vi "Right Prim.vi"() -> ()   [LabVIEW 2013]
uses:
  Goal.ctl
  <vilib>/Analysis/Matrix/Datatypes/RealMatrix.ctl
  ROS/Code/SubVIs/BaxterSide.ctl
  Baxter Examples/Arm Globals.vi
  <vilib>/Analysis/Matrix/NI_Matrix.lvlib
panel:
  out "Q size 2":i32
  in  "Zero V 2":bool
  in  "L: Home":bool caption="Home"
  in  "L: End":bool caption="Abort"
  in  "L: Pause":bool caption="Pause"
  out "L: Status":string caption="Prim Status"
  out "L: Cmd":cluster{string, "Joints":dbl[]}
  in  "Use Sparse":bool=TRUE
  out "Q size":i32
  in  "Zero V":bool
  in  "R: Home":bool caption="Home"
  in  "R: End":bool caption="Abort"
  in  "R: Pause":bool caption="Pause"
  in  "stop":bool
  out "Status":string caption="Prim Status"
  out "R: Cmd":cluster{string, "Joints":dbl[]}
  # "Right"
  # "Left"
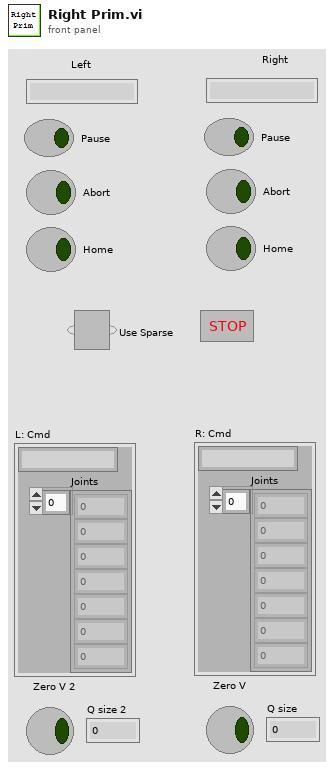
[diagram p1: front panel]
types:
  T1 = typedef "Goal.ctl" = cluster{"Segment":dbl, "T Matrix":T2, "Joints":dbl[], "Label":string, "Joint Motion":bool}
  T2 = typedef "NI_Matrix.lvlib/RealMatrix.ctl" = dbl[][]
  T3 = typedef "BaxterSide.ctl" = enum16{"left", "right"}
  T4 = enum32{"Position", "Velocity", "Effort", "Pause", "Repeat", "End"}
  T5 = typedef "_ROSControl.ctl" = cluster{"topic port":u16, "Node":string, "topic":string, "type":string, "node port":u32, "error ":errorcluster, "Direction":T6, "APIs":string[]}
  T6 = typedef "_ROSDirection.ctl" = enum16{"Node", "Publisher", "Subscriber", "Service Client"}
  T7 = cluster{"Joint Names":string[], "Position":dbl[], "Velocity":dbl[], "Effort":dbl[]}
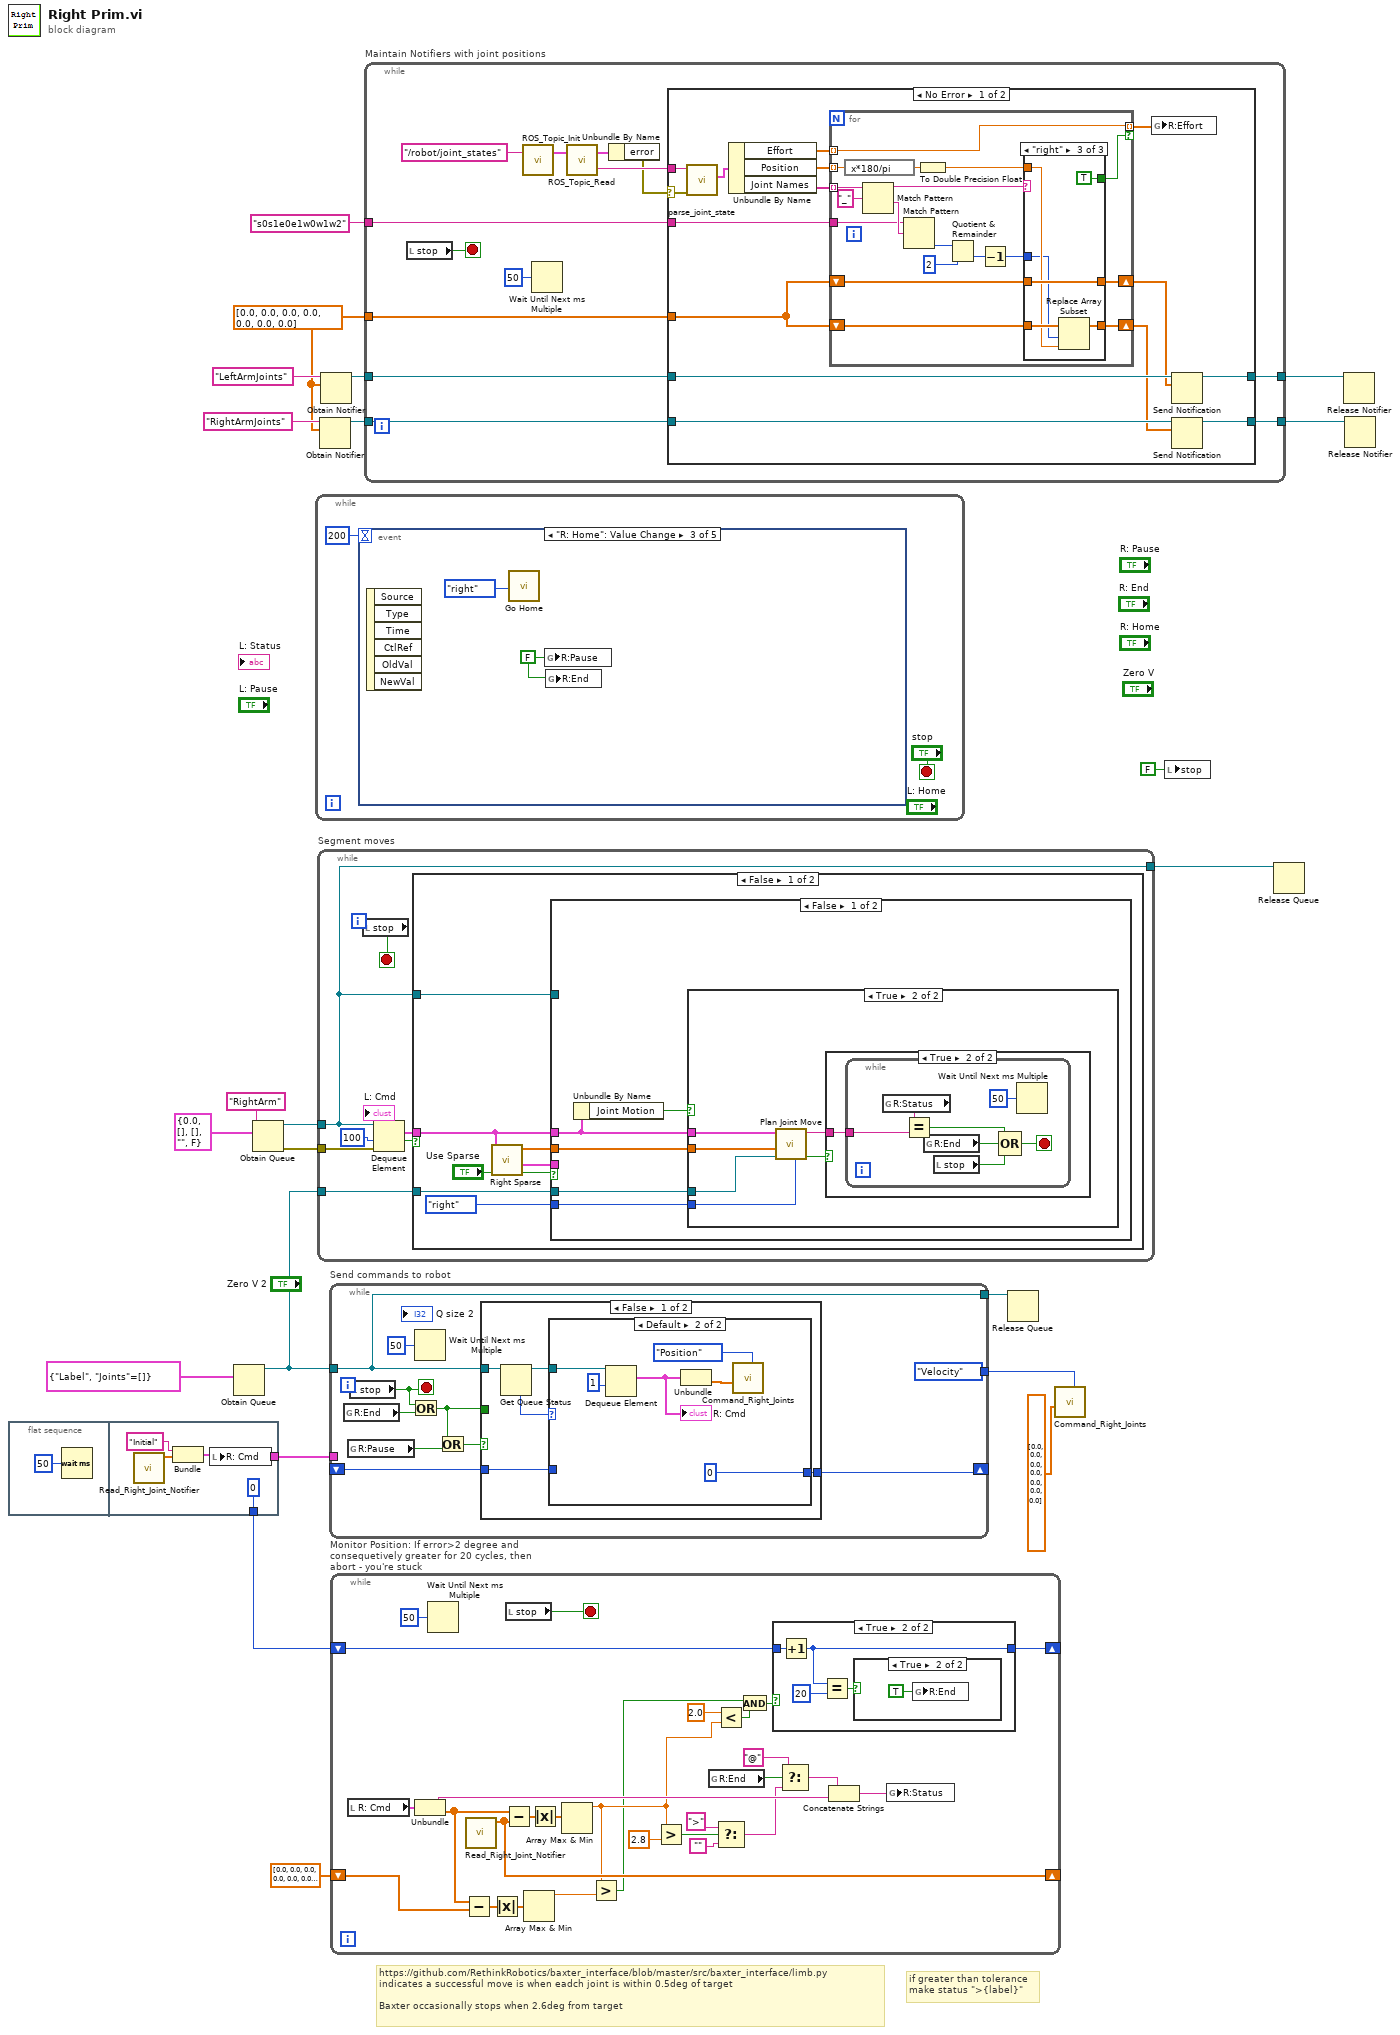
[diagram p0: block diagram]
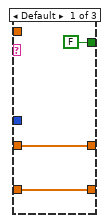
[diagram p2: hidden frame]
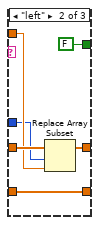
[diagram p3: hidden frame]
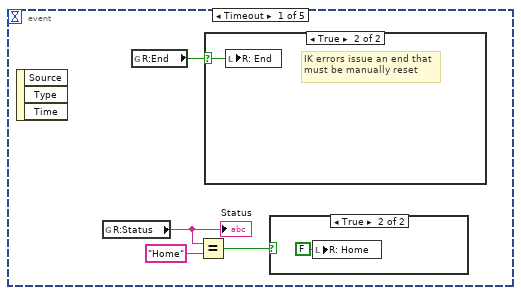
[diagram p5: hidden frame]
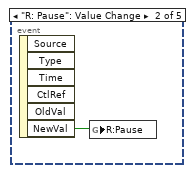
[diagram p8: hidden frame]
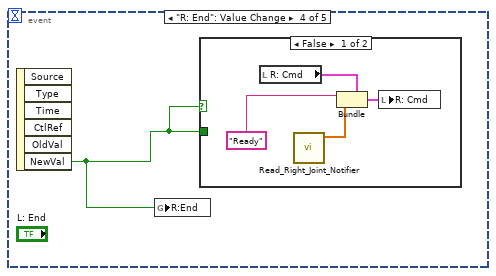
[diagram p9: hidden frame]
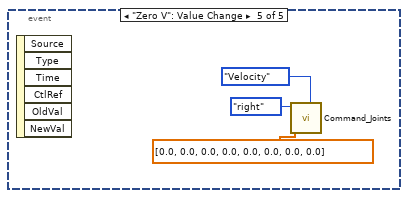
[diagram p11: hidden frame]
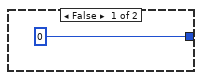
[diagram p12: hidden frame]
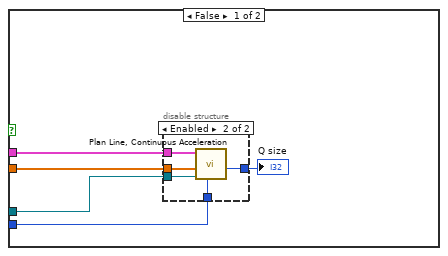
[diagram p14: hidden frame]
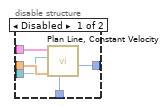
[diagram p15: hidden frame]
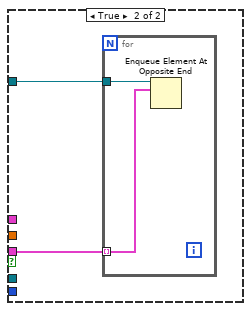
[diagram p17: hidden frame]
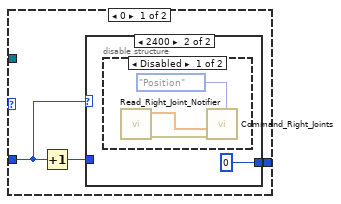
[diagram p19: hidden frame]
diagram:
  w7 = dbl[] [0.0, 0.0, 0.0, 0.0, 0.0, 0.0, 0.0]
  # "https://github.com/RethinkRobotics/baxter_interface/blob/master/src/baxter_interface/limb.py\nindicates a successful move is when eadch joint is within 0.5deg of target\n\nBaxter occasionally stops when 2.6deg from target"
  # "if greater than tolerance \nmake status \">{label}\""
  n1 = flat-sequence {
    tunnel: [w25] -> w3
    tunnel: [0] -> w2
    frame #0 {
      n2 = Wait (ms)(milliseconds to wait=u32 50) -> ()  [unwired: 1 out]
    }
    frame #1 {
      n3 = call "Read_Right_Joint_Notifier.vi"() -> ("Positions"=w26:dbl[])  [unwired: 7 in, 1 out]
      n4 = Bundle("Initial", "Positions"=w26) -> (w25:cluster{string, "Positions":dbl[]})  [unwired: 1 in]
      n5 = local write "R: Cmd"(w25) -> ()
    }
  }
  n6 = Obtain Queue(element data type=cluster{string, "Joints":dbl[]} {"Label", "Joints"=[]}) -> (queue out=w17:refnum<queue>)  [unwired: 4 in, 2 out]
  n7 = Obtain Queue(name (unnamed)="RightArm", element data type=T1 {"Segment"=0.0, "T Matrix"=[], "Joints"=[], "Label"="", "Joint Motion"=FALSE} ("Goal")) -> (queue out=w20:refnum<queue>, error out=w19:errorcluster)  [unwired: 3 in, 1 out]
  n8 = while {
    stop <- "stop" stop-if-true
    n9 = event shown="[2] \"R: Home\": Value Change" {
      selector: _ -> [_ _ _ _ _]
      dyn-events: _ -> [_ _ _ _ _]
      timeout: 200 -> [_ _ _ _ _]
      event Timeout {
        n10 = event-data() -> ()  [unwired: 1 in, 3 out]
        n11 = global read "Arm Globals.vi" "R:Status"() -> (w30:string)
        "Status" <- w30
        n12 = global read "Arm Globals.vi" "R:End"() -> (w31:bool)
        n13 = Equal?(x=w30, y="Home") -> (x = y?=w32:bool)
        n14 = case shown="True" w31 {
          selector: w31 -> [_ w34]
          frame False {
          }
          frame True {
            # "IK errors issue an end that\nmust be manually reset"
            n15 = local write "R: End"(w34) -> ()
          }
        }
        n16 = case shown="True" w32 {
          frame False {
          }
          frame True {
            n17 = local write "R: Home"(FALSE ("Home")) -> ()
          }
        }
      }
      event "R: Pause": Value Change {
        n18 = event-data() -> ("NewVal"=w36:bool)  [unwired: 1 in, 5 out]
        n19 = global write "Arm Globals.vi" "R:Pause"(w36) -> ()
      }
      event "R: Home": Value Change {
        w38 = FALSE ("R:Pause")
        n20 = event-data() -> ()  [unwired: 1 in, 6 out]
        n21 = call "Go Home.vi"("Side"=BaxterSide."right") -> ()  [unwired: 11 in]
        n22 = global write "Arm Globals.vi" "R:Pause"(w38) -> ()
        n23 = global write "Arm Globals.vi" "R:End"(w38) -> ()
      }
      event "R: End": Value Change {
        n24 = event-data() -> ("NewVal"=w39:bool)  [unwired: 1 in, 5 out]
        n25 = global write "Arm Globals.vi" "R:End"(w39) -> ()
        n26 = case shown="False" w39 {
          tunnel: w39 -> [_ _]
          frame False {
            n27 = local read "R: Cmd"() -> (w43:cluster{string, "Joints":dbl[]})
            n28 = call "Read_Right_Joint_Notifier.vi"() -> ("Positions"=w40:dbl[])  [unwired: 7 in, 1 out]
            n29 = Bundle(cluster=w43, "Ready" ("f"), "Joints"=w40) -> (w41:cluster{string, "Joints":dbl[]})
            n30 = local write "R: Cmd"(w41) -> ()
          }
          frame True {
          }
        }
      }
      event "Zero V": Value Change {
        n31 = event-data() -> ()  [unwired: 1 in, 6 out]
        n32 = call "Command_Joints.vi"("Mode"=T4."Velocity", "Arm Angles (degrees)"=dbl[] [0.0, 0.0, 0.0, 0.0, 0.0, 0.0, 0.0, 0.0] ("Joints"), "Side"=BaxterSide."right") -> ()  [unwired: 5 in, 2 out]
      }
    }
  }
  n33 = while "Segment moves" {
    tunnel: w20 -> [w47]
    tunnel: w19 -> [w50]
    tunnel: [w47] -> w18
    tunnel: w17 -> [w49]
    stop <- w48 stop-if-true
    n34 = local read "stop"() -> (w48:bool)
    n35 = Dequeue Element(queue=w47, timeout in ms (-1)=100, error in (no error)=w50) -> (element=w51:T1, timed out?=w52:bool)  [unwired: 2 out]
    n36 = case shown="False" w52 {
      tunnel: w51 -> [w58 _]
      tunnel: w49 -> [w61 _]
      tunnel: w47 -> [w60 _]
      frame False {
        n37 = call "Right Sparse.vi"("Use Sparse"="Use Sparse", "Goal"=w58) -> ("Use Backfill"=w55:bool, "Backfill"=w54:T1[], "Current"=w57:dbl[])  [unwired: 7 in]
        n38 = case shown="False" w55 {
          tunnel: w61 -> [w66 _]
          tunnel: w60 -> [_ w96]
          tunnel: BaxterSide."right" ("Side") -> [w64 _]
          tunnel: w58 -> [w63 _]
          tunnel: w57 -> [w62 _]
          tunnel: w54 -> [_ w97]
          frame False {
            n39 = Unbundle By Name(w63) -> ("Joint Motion"=w65:bool)
            n40 = case shown="True" w65 {
              tunnel: w66 -> [w68 w85]
              tunnel: w63 -> [w70 w87]
              tunnel: w62 -> [w69 w86]
              tunnel: w64 -> [w67 w84]
              frame False {
                n41 = disable-structure shown="Enabled" {
                  disable-tunnel: [w76 w81] -> w71
                  disable-tunnel: w69 -> [w75 w78]
                  disable-tunnel: w67 -> [w74 w79]
                  disable-tunnel: w70 -> [w73 w80]
                  disable-tunnel: w68 -> [w72 w77]
                  frame Disabled {
                    n42 = call "Plan Line, Constant Velocity.vi"("Side"=w74, "Joints"=w75, "queue"=w72, "Goal"=w73) -> ("Q size"=w76:i32)  [unwired: 7 in]
                  }
                  frame Enabled {
                    n43 = call "Plan Line, Continuous Acceleration.vi"("Side"=w79, "queue"=w77, "Joints"=w78, "Goal"=w80) -> ("Q size"=w81:i32)  [unwired: 7 in]
                  }
                }
                "Q size" <- w71
              }
              frame True {
                # "Joint motion command"
                n44 = call "Plan Joint Move.vi"("Side"=w84, "queue"=w85, "Joints"=w86, "Goal"=w87) -> ("0 Speed?"=w82:bool, "Label"=w83:string)  [unwired: 6 in]
                n45 = case shown="True" w82 {
                  tunnel: w83 -> [_ w88]
                  frame False {
                  }
                  frame True {
                    # "Wait for completion of\nzero speed motions"
                    n46 = while {
                      tunnel: w88 -> [w91]
                      stop <- w93 stop-if-true
                      n47 = global read "Arm Globals.vi" "R:Status"() -> (w90:string)
                      n48 = Equal?(x=w90, y=w91) -> (x = y?=w89:bool)
                      n49 = global read "Arm Globals.vi" "R:End"() -> (w94:bool)
                      n50 = local read "stop"() -> (w95:bool)
                      n51 = Compound Arithmetic op=OR(w89, w94, w95) -> (w93:bool)
                      n52 = Wait Until Next ms Multiple(millisecond multiple=u32 50) -> ()  [unwired: 1 out]
                    }
                  }
                }
              }
            }
          }
          frame True {
            n53 = for {
              tunnel: w97 -> [w98] mode=indexing
              tunnel: w96 -> [w99]
              n54 = Enqueue Element At Opposite End(queue=w99, element=w98) -> ()  [unwired: 2 in, 3 out]
            }
          }
        }
      }
      frame True {
      }
    }
  }
  n55 = Obtain Notifier(name (unnamed)="RightArmJoints", notification data type=w7) -> (notifier out=w8:refnum<notifier>)  [unwired: 2 in, 2 out]
  n56 = Obtain Notifier(name (unnamed)="LeftArmJoints", notification data type=w7) -> (notifier out=w9:refnum<notifier>)  [unwired: 2 in, 2 out]
  n57 = while "Send commands to robot" {
    tunnel: w17 -> [w104]
    tunnel: [w104] -> w22
    shift-right: [w103] -> _
    shift-left: _ -> [w102]
    tunnel: [enum32{"Position", "Velocity", "Effort"}."Velocity" ("Mode")] -> w13
    tunnel: w3 -> [_]
    stop <- w101 stop-if-true
    n58 = global read "Arm Globals.vi" "R:End"() -> (w106:bool)
    n59 = global read "Arm Globals.vi" "R:Pause"() -> (w108:bool)
    n60 = local read "stop"() -> (w101:bool)
    n61 = Or(x=w101, y=w106) -> (x .or. y?=w105:bool)
    n62 = Wait Until Next ms Multiple(millisecond multiple=u32 50) -> ()  [unwired: 1 out]
    n63 = Or(x=w105, y=w108) -> (x .or. y?=w107:bool)
    n64 = case shown="False" w107 {
      tunnel: w104 -> [w114 w130]
      tunnel: w105 -> [_ w131]
      tunnel: [w111 w129] -> w103
      tunnel: w102 -> [w110 w129]
      frame False {
        n65 = Get Queue Status(queue=w114) -> (queue out=w113:refnum<queue>, # elements in queue=w112:i32)  [unwired: 2 in, 6 out]
        n66 = case shown="Default" w112 {
          tunnel: w113 -> [_ w127]
          tunnel: [w117 0] -> w111
          tunnel: w110 -> [w116 _]
          frame 0 {
            n67 = Increment(x=w116) -> (x+1=w115:i32)
            n68 = case shown="2400" w116 {
              tunnel: [w118 0] -> w117
              tunnel: w115 -> [w118 _]
              frame 0, Default {
              }
              frame 2400 {
                n69 = disable-structure shown="Disabled" {
                  frame Disabled {
                    n70 = call "Read_Right_Joint_Notifier.vi"() -> ("error out"=w120:errorcluster, "Positions"=w121:dbl[])  [unwired: 7 in]
                    n71 = call "Command_Right_Joints.vi"("Mode"=enum32{"Position", "Velocity", "Effort"}."Position", "error in"=w120, "Arm Angles (degrees)"=w121) -> ()  [unwired: 5 in, 2 out]
                  }
                  frame Enabled {
                  }
                }
              }
            }
          }
          frame Default {
            n72 = Dequeue Element(queue=w127, timeout in ms (-1)=1) -> (element=w126:cluster{string, "Joints":dbl[]})  [unwired: 1 in, 3 out]
            "R: Cmd" <- w126
            n73 = Unbundle(w126) -> ("Joints"=w124:dbl[])  [unwired: 1 out]
            n74 = call "Command_Right_Joints.vi"("Mode"=T4."Position", "Arm Angles (degrees)"=w124) -> ()  [unwired: 6 in, 2 out]
          }
        }
      }
      frame True {
        n75 = case shown="True" w131 {
          tunnel: w130 -> [_ w134]
          frame False {
          }
          frame True {
            n76 = Flush Queue(queue=w134) -> ()  [unwired: 1 in, 3 out]
            n77 = call "Command_Right_Joints.vi"("Mode"=enum32{"Position", "Velocity", "Effort"}."Velocity", "Arm Angles (degrees)"=dbl[] [0.0, 0.0, 0.1318359373493555, 0.0, 0.0, 0.0, 0.0] ("Joints")) -> ()  [unwired: 6 in, 2 out]
          }
        }
      }
    }
  }
  n78 = while "Monitor Position: If error>2 degree and consequetively greater for 20 cycles, then abort - you're stuck" {
    shift-right: [w159] -> _
    shift-left: w2 -> [w158]
    shift-right: [w142] -> _
    shift-left: dbl[] [0.0, 0.0, 0.0, 0.0, 0.0, 0.0, 0.0] ("Positions") -> [w139]
    stop <- w156 stop-if-true
    n79 = local read "R: Cmd"() -> (w157:cluster{string, "Joints":dbl[]})
    n80 = Unbundle(w157) -> (w150:string, "Joints"=w140:dbl[])
    n81 = Wait Until Next ms Multiple(millisecond multiple=u32 50) -> ()  [unwired: 1 out]
    n82 = Subtract(x=w140, y=w139) -> (x-y=w138:dbl[])
    n83 = call "Read_Right_Joint_Notifier.vi"() -> ("Positions"=w142:dbl[])  [unwired: 7 in, 1 out]
    n84 = Absolute Value(x=w138) -> (abs(x)=w141:dbl[])
    n85 = Subtract(x=w140, y=w142) -> (x-y=w162:dbl[])
    n86 = local read "stop"() -> (w156:bool)
    n87 = Array Max & Min(array=w141) -> (max value=w137:dbl)  [unwired: 3 out]
    n88 = Absolute Value(x=w162) -> (abs(x)=w155:dbl[])
    n89 = Array Max & Min(array=w155) -> (max value=w136:dbl)  [unwired: 3 out]
    n90 = Greater?(x=w136, y=w137) -> (0:w135:bool)
    n91 = Greater?(x=w136, y=2.8) -> (0:w153:bool)
    n92 = global read "Arm Globals.vi" "R:End"() -> (w146:bool)
    n93 = Less?(x=2.0, y=w136) -> (x < y?=w148:bool)
    n94 = Select(t=">", s=w153, f="") -> (s? t:f=w144:string)
    n95 = And(x=w135, y=w148) -> (x .and. y?=w147:bool)
    n96 = case shown="True" w147 {
      tunnel: [0 w166] -> w159
      tunnel: w158 -> [_ w167]
      frame False {
      }
      frame True {
        n97 = Increment(x=w167) -> (x+1=w166:i32)
        n98 = Equal?(x=w166, y=20) -> (x = y?=w164:bool)
        n99 = case shown="True" w164 {
          frame False {
          }
          frame True {
            n100 = global write "Arm Globals.vi" "R:End"(TRUE ("R:End")) -> ()
          }
        }
      }
    }
    n101 = Select(t="@" ("string"), s=w146, f=w144) -> (s? t:f=w143:string)
    n102 = Concatenate Strings(w143, w150) -> (w149:string)
    n103 = global write "Arm Globals.vi" "R:Status"(w149) -> ()
  }
  n104 = while "Maintain Notifiers with joint positions" {
    tunnel: w9 -> [w176]
    tunnel: w8 -> [w174]
    tunnel: w7 -> [w178]
    tunnel: [w175] -> w5
    tunnel: [w173] -> w6
    tunnel: "s0s1e0e1w0w1w2" -> [w171]
    stop <- w169 stop-if-true
    n105 = local read "stop"() -> (w169:bool)
    n106 = call "ROS_Topic_Init.vi"("topic"="/robot/joint_states") -> ("ROS out"=w180:T5)  [unwired: 2 in]
    n107 = Wait Until Next ms Multiple(millisecond multiple=u32 50 ("milliseconds to wait")) -> ()  [unwired: 1 out]
    n108 = call "ROS_Topic_Read.vi"("ROS in"=w180) -> ("Reply"=w172:string, "ROS out"=w179:T5)  [unwired: 1 in]
    n109 = Unbundle By Name(w179) -> ("error"=w170:errorcluster)
    n110 = case shown="No Error" w170 {
      selector: w170 -> [w185 _]
      tunnel: w178 -> [w196 _]
      tunnel: w176 -> [w195 w231]
      tunnel: [w193 w231] -> w175
      tunnel: w174 -> [w192 w230]
      tunnel: [w191 w230] -> w173
      tunnel: w172 -> [w190 _]
      tunnel: w171 -> [w186 _]
      frame No Error {
        n111 = call "parse_joint_state.vi"("error in"=w185, "msg in"=w190) -> ("ROS Joint States"=w189:T7)  [unwired: 2 in, 3 out]
        n112 = Unbundle By Name(w189) -> ("Effort"=w183:dbl[], "Position"=w188:dbl[], "Joint Names"=w187:string[])
        n113 = for {
          shift-right: [w214] -> w194
          shift-left: w196 -> [w213]
          shift-right: [w211] -> w184
          shift-left: w196 -> [w212]
          tunnel: w187 -> [w207] mode=indexing
          tunnel: w188 -> [w210] mode=indexing
          tunnel: w186 -> [w200]
          tunnel: w183 -> [w198] mode=indexing
          tunnel: [w198] -> w182 mode=indexing if=w197
          n114 = expression code="x*180/pi"(w210) -> (w209:dbl)
          n115 = Match Pattern(string=w207, regular expression="_") -> (before substring=w201:string, after substring=w205:string)  [unwired: 1 in, 2 out]
          n116 = Match Pattern(string=w200, regular expression=w205) -> (offset past match=w204:i32)  [unwired: 1 in, 3 out]
          n117 = To Double Precision Float(number=w209) -> (double precision float=w208:dbl)
          n118 = Quotient & Remainder(x=w204, y=2) -> (floor(x/y)=w202:i32)  [unwired: 1 out]
          n119 = Decrement(x=w202) -> (x-1=w199:i32)
          n120 = case shown="\"right\"" w201 {
            tunnel: [w217 w221 w229] -> w214
            tunnel: w213 -> [w217 w222 w229]
            tunnel: w208 -> [_ w220 w226]
            tunnel: w212 -> [w216 w223 w227]
            tunnel: [w216 w223 w228] -> w211
            tunnel: w199 -> [_ w219 w225]
            tunnel: [FALSE FALSE TRUE] -> w197
            frame Default {
            }
            frame "left" {
              n121 = Replace Array Subset(array=w222, new element=w220, index=w219) -> (w221:dbl[])
            }
            frame "right" {
              n122 = Replace Array Subset(array=w227, new element=w226, index=w225) -> (w228:dbl[])
            }
          }
        }
        n123 = global write "Arm Globals.vi" "R:Effort"(w182) -> ()
        n124 = Send Notification(notification=w194, notifier=w195) -> (notifier out=w193:refnum<notifier>)  [unwired: 1 in, 1 out]
        n125 = Send Notification(notification=w184, notifier=w192) -> (notifier out=w191:refnum<notifier>)  [unwired: 1 in, 1 out]
      }
      frame Error {
      }
    }
  }
  n126 = Release Queue(queue=w22) -> ()  [unwired: 2 in, 3 out]
  n127 = call "Command_Right_Joints.vi"("Mode"=w13, "Arm Angles (degrees)"=dbl[] [0.0, 0.0, 0.0, 0.0, 0.0, 0.0, 0.0]) -> ()  [unwired: 6 in, 2 out]
  n128 = local write "stop"(FALSE ("stop")) -> ()
  n129 = Release Queue(queue=w18) -> ()  [unwired: 2 in, 3 out]
  n130 = Release Notifier(notifier=w5) -> ()  [unwired: 2 in, 3 out]
  n131 = Release Notifier(notifier=w6) -> ()  [unwired: 2 in, 3 out]
